vi "数据写入database.vi"(9 "data":variant, 10 "columns":string[](array[string]), 11 "table":string) -> (1 "error out":errorcluster)   [LabVIEW 2016, in "斯坦道CODMn.lvlib"]
uses:
  <vilib>/addons/database/Connection.llb/DB Tools Open Connec (String).vi
  <vilib>/addons/database/Connection.llb/Conn Execute.vi
  <vilib>/addons/database/Recordset.llb/Rec Destroy - Connection.vi
  <vilib>/addons/database/Recordset.llb/Rec Fetch Recordset Data (R).vi
  <vilib>/addons/database/NI_Database_API.lvlib
panel:
  out "为空？":bool
  in  "error in (no error)":errorcluster
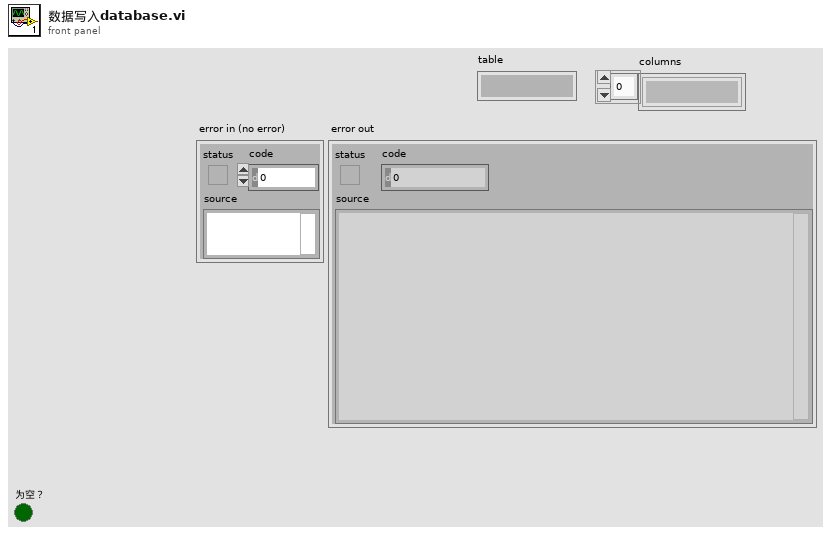
[diagram p1: front panel]
types:
  T1 = cluster{"时间":timestamp, "测量模式":string, "数据类型":string, "检测值":sgl, "单位":string, "数据标识":string, "因子编码":string, "标样参考值":sgl, "ORP-A":sgl, "ORP-B":sgl, "ORP-K":sgl, "COD滴定值":sgl, "高锰酸钾滴定数":sgl, "温度":sgl, "序列号":string, "量程":sgl, "LastTime":timestamp}
  T2 = typedef "NI_Database_API.lvlib/Conn ObjectReference.ctl" = refnum<k1>
  T3 = typedef "NI_Database_API.lvlib/Rec ObjectReference.ctl" = refnum<k1>
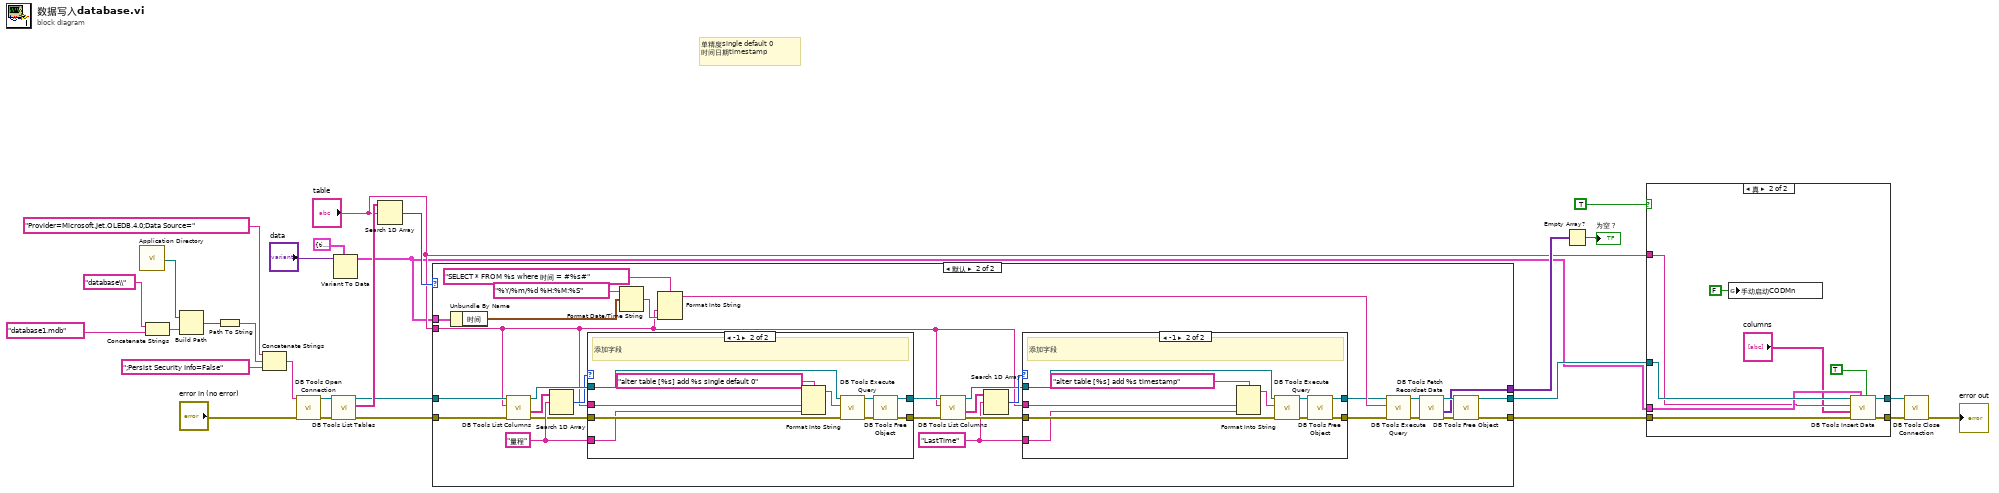
[diagram p0: block diagram]
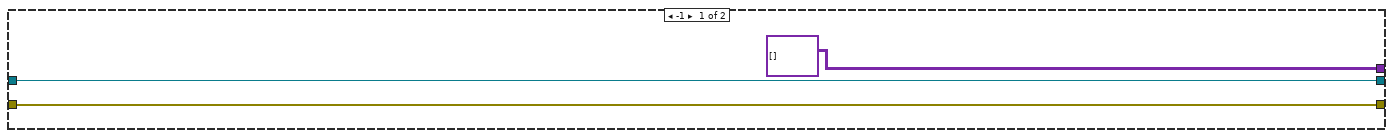
[diagram p2: hidden frame]
diagram:
  # "单精度single default 0\n时间日期timestamp"
  n1 = call <vilib>:"Application Directory.vi"() -> ("Application Directory"=w3:path)
  n2 = Concatenate Strings("database\\" ("condition"), "database1.mdb" ("字符串")) -> (w22:string)
  n3 = Build Path(base path=w3, name or relative path=w22) -> (appended path=w27:path)
  n4 = Path To String(path=w27) -> (string=w26:string)
  n5 = Concatenate Strings("Provider=Microsoft.Jet.OLEDB.4.0;Data Source=" ("condition"), w26, ";Persist Security Info=False" ("condition")) -> (w24:string)
  n6 = call-poly <vilib>:"DB Tools Open Connection.vi"("error in (no error)"="error in (no error)", "connection information"=w24) -> ("error out"=w20:errorcluster, "connection reference"=w21:T2)  [unwired: 6 in]
  n7 = call <vilib>:"DB Tools List Tables.vi"("error in (no error)"=w20, "connection reference"=w21) -> ("error out"=w14:errorcluster, "tables"=w19:string[], "connection reference out"=w15:T2)  [unwired: 3 in]
  n8 = Variant To Data(type=T1 {"时间"=timestamp(0 s since 1904-01-01), "测量模式"="", "数据类型"="", "检测值"=0.0, "单位"="", "数据标识"="", "因子编码"="", "标样参考值"=0.0, "ORP-A"=0.0, "ORP-B"=0.0, "ORP-K"=0.0, "COD滴定值"=0.0, "高锰酸钾滴定数"=0.0, "温度"=0.0, "序列号"="", "量程"=0.0, "LastTime"=timestamp(0 s since 1904-01-01)} ("data"), Variant="data") -> (data=w4:T1)  [unwired: 1 in, 1 out]
  n9 = Search 1D Array(1D array=w19, element="table") -> (index of element=w16:i32)  [unwired: 1 in]
  n10 = case shown="默认" w16 {
    tunnel: [variant[][] [] ("recordset data") w43] -> w13
    tunnel: [w31 w57] -> w12
    tunnel: [w30 w56] -> w11
    tunnel: w15 -> [w31 w45]
    tunnel: w14 -> [w30 w44]
    tunnel: "table" -> [_ w34]
    tunnel: w4 -> [_ w51]
    frame -1 {
    }
    frame Default {
      w38 = "LastTime" ("元素")
      w49 = "量程" ("元素")
      n11 = Unbundle By Name(w51) -> ("时间"=w54:timestamp)
      n12 = call <vilib>:"DB Tools List Columns.vi"("error in (no error)"=w44, "table"=w34, "connection reference"=w45) -> ("error out"=w47:errorcluster, "columns"=w48:string[], "connection reference out"=w50:T2)  [unwired: 1 in, 1 out]
      n13 = Search 1D Array(1D array=w48, element=w49) -> (index of element=w46:i32)  [unwired: 1 in]
      n14 = case shown="-1" w46 {
        tunnel: w50 -> [w75 w83]
        tunnel: w47 -> [w74 w82]
        tunnel: w49 -> [_ w80]
        tunnel: [w75 w78] -> w36
        tunnel: [w74 w77] -> w35
        tunnel: w34 -> [_ w76]
        frame 0, Default {
        }
        frame -1 {
          # "添加字段"
          n15 = Format Into String(format string="alter table [%s] add %s single default 0", w76, w80) -> (resulting string=w79:string)  [unwired: 2 in, 1 out]
          n16 = call-poly <vilib>:"DB Tools Execute Query.vi"("error in (no error)"=w82, "SQL query"=w79, "connection reference"=w83) -> ("error out"=w84:errorcluster, "recordset reference"=w85:T3)  [unwired: 5 in]
          n17 = call-poly <vilib>:"DB Tools Free Object.vi"("error in (no error)"=w84, "recordset reference"=w85) -> ("error out"=w77:errorcluster, "connection reference"=w78:T2)  [unwired: 8 in]
        }
      }
      n18 = Format Date/Time String(time format string (%c)="%Y/%m/%d %H:%M:%S" ("时间格式字符串(%c)"), seconds (now)=w54) -> (date/time string=w52:string)  [unwired: 1 in]
      n19 = Format Into String(format string="SELECT * FROM %s where 时间 = #%s#" ("格式字符串"), w34, w52) -> (resulting string=w55:string)  [unwired: 2 in, 1 out]
      n20 = call <vilib>:"DB Tools List Columns.vi"("error in (no error)"=w35, "table"=w34, "connection reference"=w36) -> ("error out"=w40:errorcluster, "columns"=w39:string[], "connection reference out"=w37:T2)  [unwired: 1 in, 1 out]
      n21 = Search 1D Array(1D array=w39, element=w38) -> (index of element=w41:i32)  [unwired: 1 in]
      n22 = case shown="-1" w41 {
        tunnel: w37 -> [w63 w71]
        tunnel: w40 -> [w62 w70]
        tunnel: w38 -> [_ w68]
        tunnel: [w63 w66] -> w33
        tunnel: [w62 w65] -> w32
        tunnel: w34 -> [_ w64]
        frame 0, Default {
        }
        frame -1 {
          # "添加字段"
          n23 = Format Into String(format string="alter table [%s] add %s timestamp", w64, w68) -> (resulting string=w67:string)  [unwired: 2 in, 1 out]
          n24 = call-poly <vilib>:"DB Tools Execute Query.vi"("error in (no error)"=w70, "SQL query"=w67, "connection reference"=w71) -> ("error out"=w72:errorcluster, "recordset reference"=w73:T3)  [unwired: 5 in]
          n25 = call-poly <vilib>:"DB Tools Free Object.vi"("error in (no error)"=w72, "recordset reference"=w73) -> ("error out"=w65:errorcluster, "connection reference"=w66:T2)  [unwired: 8 in]
        }
      }
      n26 = call-poly <vilib>:"DB Tools Execute Query.vi"("error in (no error)"=w32, "SQL query"=w55, "connection reference"=w33) -> ("error out"=w58:errorcluster, "recordset reference"=w61:T3)  [unwired: 5 in]
      n27 = call-poly <vilib>:"DB Tools Fetch Recordset Data.vi"("error in (no error)"=w58, "recordset reference"=w61) -> ("error out"=w59:errorcluster, "recordset data"=w43:variant[][], "recordset reference out"=w60:T3)  [unwired: 3 in]
      n28 = call-poly <vilib>:"DB Tools Free Object.vi"("error in (no error)"=w59, "recordset reference"=w60) -> ("error out"=w56:errorcluster, "connection reference"=w57:T2)  [unwired: 8 in]
    }
  }
  n29 = Empty Array?(array=w13) -> (empty?=→"为空？":bool)
  n30 = case shown="真" TRUE {
    tunnel: "table" -> [_ w90]
    tunnel: w4 -> [_ w91]
    tunnel: w11 -> [w86 w96]
    tunnel: w12 -> [w87 w95]
    tunnel: [w87 w93] -> w18
    tunnel: [w86 w92] -> w17
    frame False {
    }
    frame True {
      n31 = global write "CODMN外部API.vi" "手动启动CODMn"(FALSE ("手动启动CODMn")) -> ()
      n32 = call <vilib>:"DB Tools Insert Data.vi"("create table? (F)"=TRUE, "data"=w91, "error in (no error)"=w96, "columns"="columns", "table"=w90, "connection reference"=w95) -> ("error out"=w92:errorcluster, "connection reference out"=w93:T2)  [unwired: 4 in]
    }
  }
  n33 = call <vilib>:"DB Tools Close Connection.vi"("error in (no error)"=w17, "connection reference"=w18) -> ("error out"=→"error out":errorcluster)  [unwired: 5 in]
